vi "FGV Pre Test Daten.vi"(0 "Daten/Ergebnisse":T1, 7 "T90 Konfig Daten":T2={"Bearbeiter:"="", "Messgerät:"="", "Seriennummer:"="", "Modus"=0, "Pfad:"=path "D:/IAG_Data/Log", "Textname:"="", "N2 Aufschaltzeit:"=120.0, "Flow weighted mean:"=120.0} caption="Drift Konfig Daten" {"Flow weighted mean:" min=10.0; "N2 Aufschaltzeit:" min=10.0; "Modus" items=["Measure", "Cal Gas to Samplepoint"]}, 11 "error in (no error)":errorcluster caption="Fehler (Eingang, kein Fehler)", 13 "Aktion":T4) -> (2 "PDF Pfad":path, 4 "Daten/Ergebnisse":T1, 8 "T90 Konfig Daten 2":T2={"Bearbeiter:"="", "Messgerät:"="", "Seriennummer:"="", "Modus"=0, "Pfad:"=path "D:/IAG_Data/Log", "Textname:"="", "N2 Aufschaltzeit:"=120.0, "Flow weighted mean:"=120.0} caption="Drift Konfig Daten" {"Flow weighted mean:" min=10.0; "N2 Aufschaltzeit:" min=10.0; "Modus" items=["Measure", "Cal Gas to Samplepoint"]}, 15 "error out":errorcluster caption="Fehler (Ausgang)")   [LabVIEW 2020, in "EPA 1065.lvlib" / "Pre-test verification 1065-520.lvlib"]
uses:
  Pre-test verification 1065-520.lvlib
  Pre Konfig Daten.ctl
  Modus Pre Test.ctl
  Aktion FGV Pre Test Daten.ctl
  Pre Werte.ctl
  Linearisierung V2/Protokoll/Protokoll.lvlib
  Allgemein/allgemeine Sub-VIs.lvlib
panel:
  # "ppm"
  # "sec."
  # "ppm"
  # "sec."
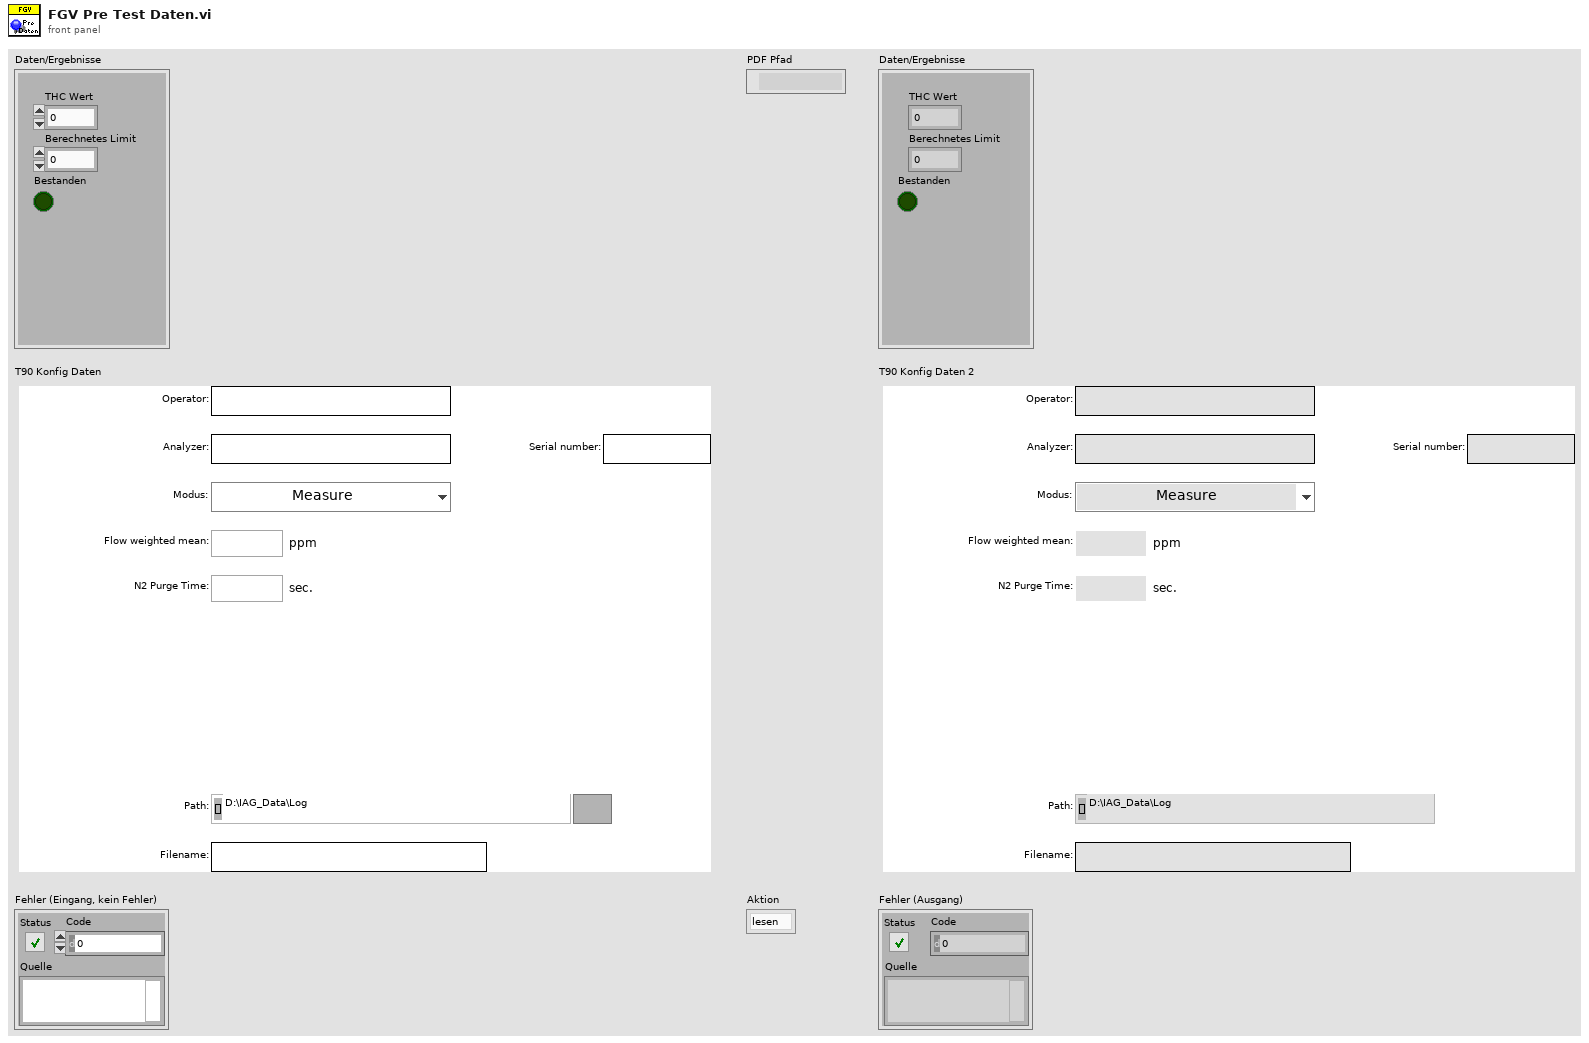
[diagram p1: front panel]
types:
  T1 = typedef "EPA 1065.lvlib/Pre-test verification 1065-520.lvlib/Pre Werte.ctl" = cluster{"THC Wert":dbl, "Berechnetes Limit":dbl, "Bestanden":bool}
  T2 = typedef "EPA 1065.lvlib/Pre-test verification 1065-520.lvlib/Pre Konfig Daten.ctl" = cluster{"Bearbeiter:":string, "Messgerät:":string, "Seriennummer:":string, "Modus":T3, "Pfad:":path, "Textname:":string, "N2 Aufschaltzeit:":dbl, "Flow weighted mean:":dbl}
  T3 = typedef "EPA 1065.lvlib/Pre-test verification 1065-520.lvlib/Modus Pre Test.ctl" = u16
  T4 = typedef "EPA 1065.lvlib/Pre-test verification 1065-520.lvlib/Aktion FGV Pre Test Daten.ctl" = enum16{"lesen", "Konfig Daten", "PDF einstellen", "laden", "speichern", "Werte schreiben", "Auswerten"}
  T5 = enum16{"open", "replace", "create", "open or create", "replace or create", "replace or create with confirmation"}
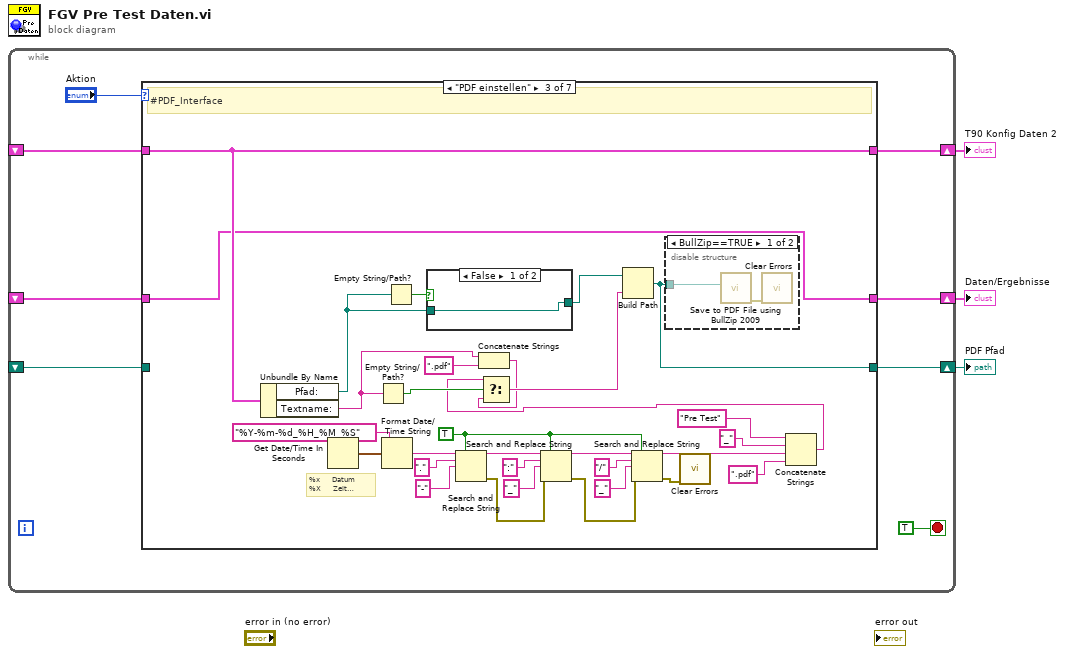
[diagram p0: block diagram]
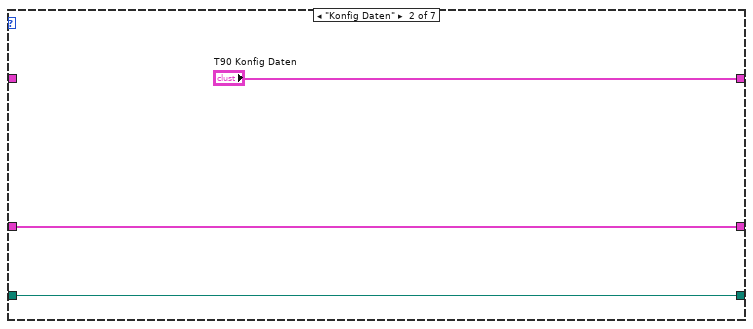
[diagram p3: hidden frame]
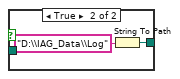
[diagram p5: hidden frame]
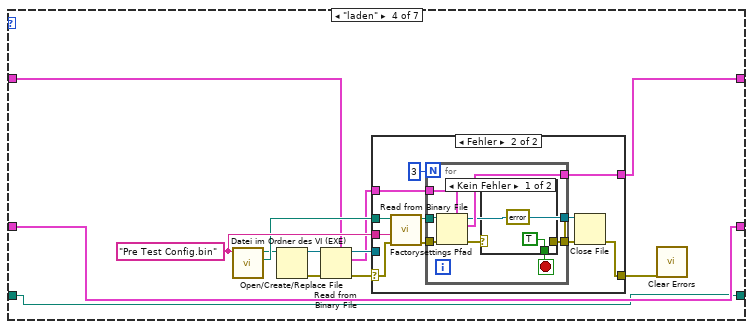
[diagram p6: hidden frame]
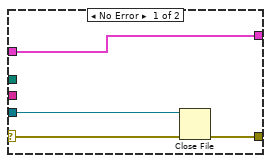
[diagram p7: hidden frame]
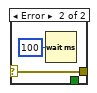
[diagram p8: hidden frame]
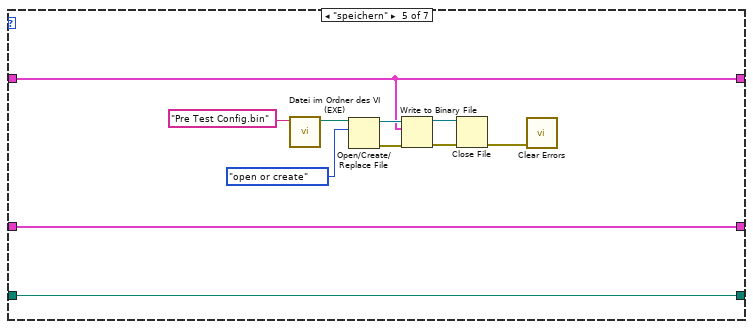
[diagram p9: hidden frame]
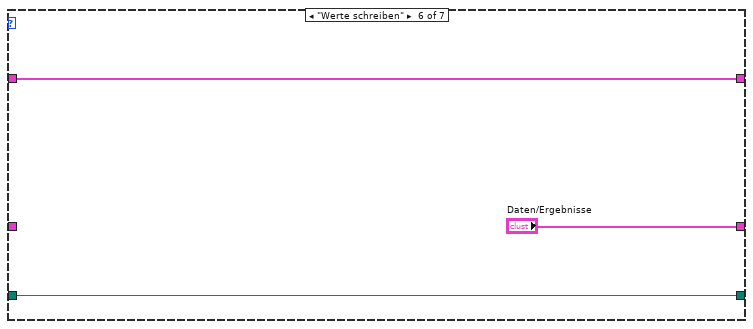
[diagram p10: hidden frame]
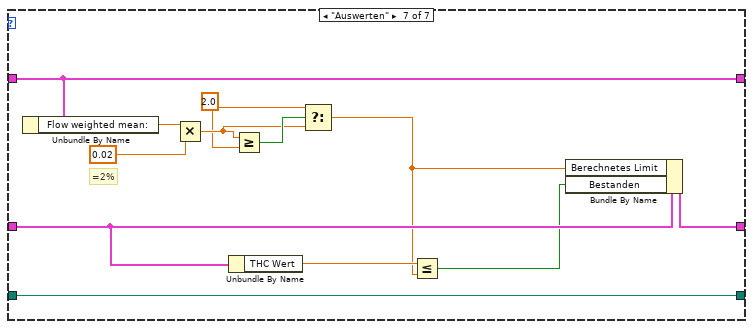
[diagram p11: hidden frame]
diagram:
  n1 = while {
    shift-right: [w9] -> w3
    shift-left: _ -> [w8]
    shift-right: [w7] -> w2
    shift-left: _ -> [w6]
    shift-right: [w5] -> w1
    shift-left: _ -> [w4]
    stop <- TRUE stop-if-true
    n2 = case shown="\"PDF einstellen\"" "Aktion" {
      tunnel: [w14 "T90 Konfig Daten" w48 w56 w97 w107 w119] -> w9
      tunnel: w8 -> [w14 _ w48 w57 w97 w107 w119]
      tunnel: [w13 w16 w22 w55 w96 "Daten/Ergebnisse" w113] -> w7
      tunnel: w6 -> [w13 w16 w22 w55 w96 _ w112]
      tunnel: [w12 w15 w18 w54 w94 w105 w108] -> w5
      tunnel: w4 -> [w12 w15 _ w54 w94 w105 w108]
      frame "lesen", Default {
      }
      frame "Konfig Daten" {
      }
      frame "PDF einstellen" {
        w39 = TRUE ("Alle ersetzen? (F)")
        # "%x      Datum\n%X      Zeit (h:m:s)"
        # "#PDF_Interface"
        n3 = Unbundle By Name(w48) -> ("Pfad:"=w24:path, "Textname:"=w20:string)
        n4 = Get Date/Time In Seconds() -> (seconds since 1Jan1904=w47:timestamp)
        n5 = Empty String/Path?(string/path=w20) -> (empty?=w27:bool)
        n6 = Format Date/Time String(time format string (%c)="%Y-%m-%d_%H_%M_%S" ("Zeitformatierungs-String (%c)"), seconds (now)=w47) -> (date/time string=w46:string)  [unwired: 1 in]
        n7 = Empty String/Path?(string/path=w24) -> (empty?=w28:bool)
        n8 = case shown="False" w28 {
          tunnel: [w51 w52] -> w23
          tunnel: w24 -> [w51 _]
          frame False {
          }
          frame True {
            n9 = String To Path(string="D:\\IAG_Data\\Log" ("Pfad")) -> (path=w52:path)
          }
        }
        n10 = Search and Replace String(replace all?=w39, input string=w46, search string="." ("Such-String"), replace string="-" ("String ersetzen(\"\")")) -> (result string=w45:string, error out=w42:errorcluster)  [unwired: 4 in, 2 out]
        n11 = Concatenate Strings(w20, ".pdf" ("String")) -> (w19:string)
        n12 = Search and Replace String(replace all?=w39, input string=w45, search string=":" ("Such-String"), replace string="_" ("String ersetzen(\"\")"), error in=w42) -> (result string=w44:string, error out=w41:errorcluster)  [unwired: 3 in, 2 out]
        n13 = Search and Replace String(replace all?=w39, input string=w44, search string="/" ("Such-String"), replace string="_" ("String ersetzen(\"\")"), error in=w41) -> (result string=w43:string, error out=w40:errorcluster)  [unwired: 3 in, 2 out]
        n14 = call <vilib>:"Clear Errors.vi"("error in (no error)"=w40) -> ()  [unwired: 5 in, 2 out]
        n15 = Concatenate Strings("Pre Test" ("String"), "_", w43, ".pdf" ("String")) -> (w26:string)
        n16 = Select(t=w26, s=w27, f=w19) -> (s? t:f=w25:string)
        n17 = Build Path(base path=w23, name or relative path=w25) -> (appended path=w18:path)
        n18 = disable-structure shown="BullZip==TRUE" {
          disable-tunnel: w18 -> [w50 _]
          frame condition #0 {
            n19 = call "Save to PDF File using BullZip 2009.vi"("Save PDF File Path"=w50) -> ("error out"=w49:errorcluster)  [unwired: 10 in]
            n20 = call <vilib>:"Clear Errors.vi"("error in (no error)"=w49) -> ()  [unwired: 5 in, 2 out]
          }
          frame condition #1 (active) {
          }
        }
      }
      frame "laden" {
        w64 = "Pre Test Config.bin" ("Dateiname")
        n21 = call "Datei im Ordner des VI (EXE).vi"("Dateiname"=w64) -> ("Ordner des Haupt-VIs"=w63:path, "Dateipfad im Ordner des Haupt-VIs"=w60:path)  [unwired: 8 in, 1 out]
        n22 = Open/Create/Replace File(file path (use dialog)=w60) -> (refnum out=w58:refnum<file>, error out=w59:errorcluster)  [unwired: 5 in, 1 out]
        n23 = Read from Binary File(5:w57, 8:w59, 11:w58) -> (0:w66:errorcluster, 2:w61:T2, 3:w62:refnum<file>)  [unwired: 3 in, 1 out]
        n24 = case shown="Fehler" w66 {
          selector: w66 -> [w69 w73]
          tunnel: w63 -> [_ w74]
          tunnel: w61 -> [w70 w72]
          tunnel: [w70 w80] -> w56
          tunnel: [w67 w78] -> w65
          tunnel: w62 -> [w68 _]
          tunnel: w64 -> [_ w71]
          frame No Error {
            n25 = Close File(refnum=w68, error in=w69) -> (error out=w67:errorcluster)  [unwired: 1 out]
          }
          frame Error {
            n26 = call "Factorysettings Pfad.vi"("error in (no error)"=w73, "Dateiname"=w71, "Ordner des Haupt-VIs"=w74) -> ("error out"=w75:errorcluster, "Pfad Factorysettings"=w76:path)  [unwired: 7 in]
            n27 = for {
              N: 3 -> [_]
              tunnel: w75 -> [w87]
              tunnel: w76 -> [w86]
              tunnel: [w85] -> w80
              tunnel: [w84] -> w79
              tunnel: [w83] -> w77
              tunnel: w72 -> [w82]
              stop <- w88 stop-if-true
              n28 = Read from Binary File(5:w82, 8:w87, 11:w86) -> (0:w89:errorcluster, 2:w85:T2, 3:w83:refnum<file>)  [unwired: 3 in, 1 out]
              n29 = case shown="Kein Fehler" w89 {
                selector: w89 -> [_ w92]
                tunnel: [TRUE _] -> w88
                tunnel: [errorcluster {"status"=FALSE, "code"=0, "source"=""} ("error IO") w92] -> w84
                frame No Error {
                }
                frame Error {
                  n30 = Wait (ms)(milliseconds to wait=u32 100 ("Zu wartende ms")) -> ()  [unwired: 1 out]
                }
              }
            }
            n31 = Close File(refnum=w77, error in=w79) -> (error out=w78:errorcluster)  [unwired: 1 out]
          }
        }
        n32 = call <vilib>:"Clear Errors.vi"("error in (no error)"=w65) -> ()  [unwired: 5 in, 2 out]
      }
      frame "speichern" {
        n33 = call "Datei im Ordner des VI (EXE).vi"("Dateiname"="Pre Test Config.bin") -> ("Dateipfad im Ordner des Haupt-VIs"=w102:path)  [unwired: 8 in, 2 out]
        n34 = Open/Create/Replace File(file path (use dialog)=w102, operation (0:open)=T5."open or create" ("Operation (0:open)")) -> (refnum out=w101:refnum<file>, error out=w103:errorcluster)  [unwired: 4 in, 1 out]
        n35 = Write to Binary File(file (use dialog)=w101, data=w97, error in=w103) -> (refnum out=w100:refnum<file>, error out=w99:errorcluster)  [unwired: 3 in, 1 out]
        n36 = Close File(refnum=w100, error in=w99) -> (error out=w98:errorcluster)  [unwired: 1 out]
        n37 = call <vilib>:"Clear Errors.vi"("error in (no error)"=w98) -> ()  [unwired: 5 in, 2 out]
      }
      frame "Werte schreiben" {
      }
      frame "Auswerten" {
        w114 = 2.0 ("y")
        # "=2%"
        n38 = Unbundle By Name(w119) -> ("Flow weighted mean:"=w118:dbl)
        n39 = Multiply(x=w118, y=0.02) -> (x*y=w115:dbl)
        n40 = Unbundle By Name(w112) -> ("THC Wert"=w111:dbl)
        n41 = Greater Or Equal?(x=w115, y=w114) -> (x >= y?=w116:bool)
        n42 = Select(t=w114, s=w116, f=w115) -> (s? t:f=w110:dbl)
        n43 = Less Or Equal?(x=w111, y=w110) -> (x <= y?=w109:bool)
        n44 = Bundle By Name(cluster=w112, "Berechnetes Limit"=w110, "Bestanden"=w109) -> (w113:T1)
      }
    }
  }
  "T90 Konfig Daten 2" <- w3
  "Daten/Ergebnisse" <- w2
  "PDF Pfad" <- w1
